vi "c Vector Rotate.vi"(9 "Angle":dbl, 10 "Y":dbl, 11 "X":dbl) -> (2 "New Y":dbl, 3 "New X":dbl)   [LabVIEW 2018]
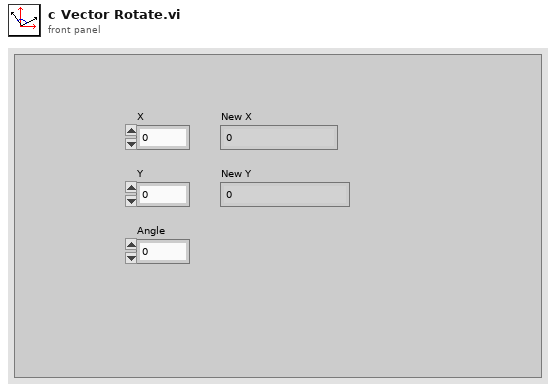
[diagram p1: front panel]
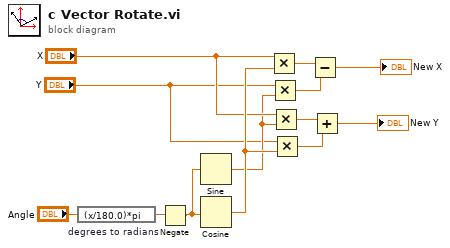
[diagram p0: block diagram]
diagram:
  n1 = expression code="(x/180.0)*pi" "degrees to radians"("Angle") -> (w2:dbl)
  n2 = Negate(x=w2) -> (-x=w1:dbl)
  n3 = Sine(x=w1) -> (sin(x)=w10:dbl)
  n4 = Cosine(x=w1) -> (cos(x)=w12:dbl)
  n5 = Multiply(x="X", y=w12) -> (x*y=w5:dbl)
  n6 = Multiply(x="Y", y=w10) -> (x*y=w6:dbl)
  n7 = Multiply(x="X", y=w10) -> (x*y=w8:dbl)
  n8 = Multiply(x="Y", y=w12) -> (x*y=w9:dbl)
  n9 = Subtract(x=w5, y=w6) -> (x-y=→"New X":dbl)
  n10 = Add(x=w8, y=w9) -> (x+y=→"New Y":dbl)
